vi "Error Converter (ErrCode or Status).vi"(0 "error code":u32, 11 "error in (no error)":errorcluster) -> (15 "error out":errorcluster)   [LabVIEW 2011, in "libMPSSE.lvlib"]
doc: "This VI generate the error description and error code from the dll error number."
uses:
  libMPSSE.lvlib
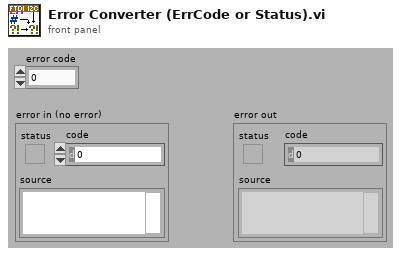
[diagram p1: front panel]
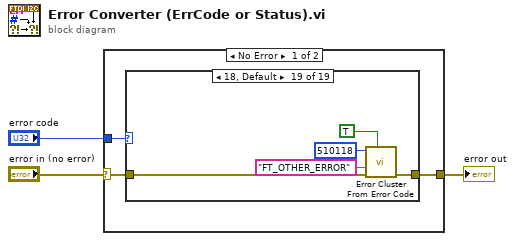
[diagram p0: block diagram]
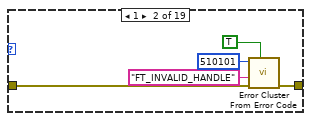
[diagram p3: hidden frame]
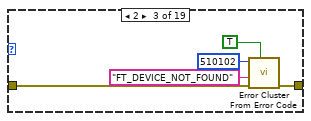
[diagram p4: hidden frame]
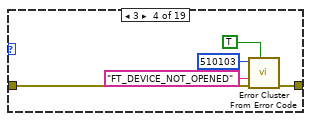
[diagram p5: hidden frame]
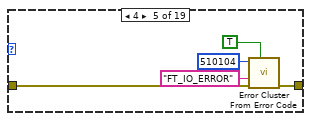
[diagram p6: hidden frame]
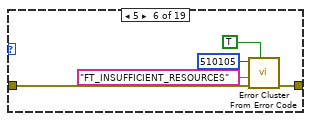
[diagram p7: hidden frame]
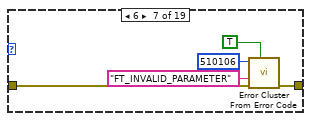
[diagram p8: hidden frame]
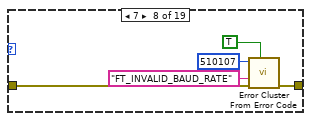
[diagram p9: hidden frame]
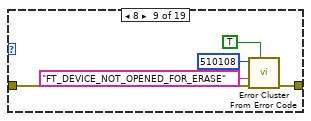
[diagram p10: hidden frame]
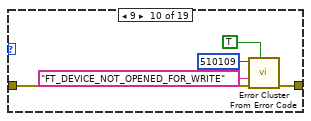
[diagram p11: hidden frame]
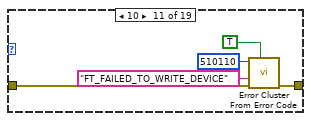
[diagram p12: hidden frame]
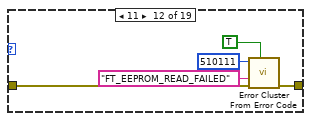
[diagram p13: hidden frame]
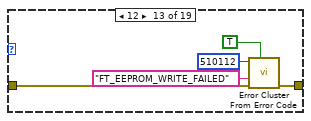
[diagram p14: hidden frame]
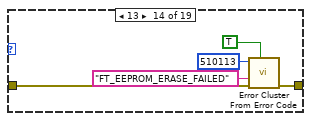
[diagram p15: hidden frame]
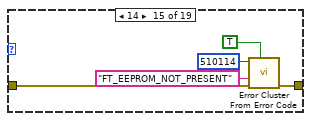
[diagram p16: hidden frame]
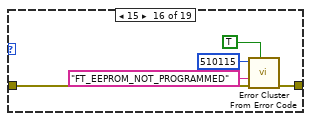
[diagram p17: hidden frame]
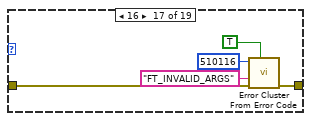
[diagram p18: hidden frame]
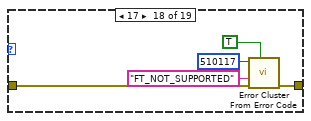
[diagram p19: hidden frame]
diagram:
  n1 = case shown="No Error" "error in (no error)" {
    selector: "error in (no error)" -> [w6 w98]
    tunnel: [w5 w98] -> w2
    tunnel: "error code" -> [w4 _]
    frame No Error {
      n2 = case shown="18, Default" w4 {
        tunnel: w6 -> [w7 w12 w17 w22 w27 w32 w37 w42 w47 w52 w57 w62 w67 w72 w77 w82 w87 w92 w97]
        tunnel: [w7 w11 w16 w21 w26 w31 w36 w41 w46 w51 w56 w61 w66 w71 w76 w81 w86 w91 w96] -> w5
        frame 0 {
        }
        frame 1 {
          n3 = call <vilib>:"Error Cluster From Error Code.vi"("show call chain? (False)"=TRUE, "error in (no error)"=w12, "error message (\"\")"="FT_INVALID_HANDLE", "error code (0)"=510101) -> ("error out"=w11:errorcluster)  [unwired: 5 in]
        }
        frame 2 {
          n4 = call <vilib>:"Error Cluster From Error Code.vi"("show call chain? (False)"=TRUE, "error in (no error)"=w17, "error message (\"\")"="FT_DEVICE_NOT_FOUND", "error code (0)"=510102) -> ("error out"=w16:errorcluster)  [unwired: 5 in]
        }
        frame 3 {
          n5 = call <vilib>:"Error Cluster From Error Code.vi"("show call chain? (False)"=TRUE, "error in (no error)"=w22, "error message (\"\")"="FT_DEVICE_NOT_OPENED", "error code (0)"=510103) -> ("error out"=w21:errorcluster)  [unwired: 5 in]
        }
        frame 4 {
          n6 = call <vilib>:"Error Cluster From Error Code.vi"("show call chain? (False)"=TRUE, "error in (no error)"=w27, "error message (\"\")"="FT_IO_ERROR", "error code (0)"=510104) -> ("error out"=w26:errorcluster)  [unwired: 5 in]
        }
        frame 5 {
          n7 = call <vilib>:"Error Cluster From Error Code.vi"("show call chain? (False)"=TRUE, "error in (no error)"=w32, "error message (\"\")"="FT_INSUFFICIENT_RESOURCES", "error code (0)"=510105) -> ("error out"=w31:errorcluster)  [unwired: 5 in]
        }
        frame 6 {
          n8 = call <vilib>:"Error Cluster From Error Code.vi"("show call chain? (False)"=TRUE, "error in (no error)"=w37, "error message (\"\")"="FT_INVALID_PARAMETER", "error code (0)"=510106) -> ("error out"=w36:errorcluster)  [unwired: 5 in]
        }
        frame 7 {
          n9 = call <vilib>:"Error Cluster From Error Code.vi"("show call chain? (False)"=TRUE, "error in (no error)"=w42, "error message (\"\")"="FT_INVALID_BAUD_RATE", "error code (0)"=510107) -> ("error out"=w41:errorcluster)  [unwired: 5 in]
        }
        frame 8 {
          n10 = call <vilib>:"Error Cluster From Error Code.vi"("show call chain? (False)"=TRUE, "error in (no error)"=w47, "error message (\"\")"="FT_DEVICE_NOT_OPENED_FOR_ERASE", "error code (0)"=510108) -> ("error out"=w46:errorcluster)  [unwired: 5 in]
        }
        frame 9 {
          n11 = call <vilib>:"Error Cluster From Error Code.vi"("show call chain? (False)"=TRUE, "error in (no error)"=w52, "error message (\"\")"="FT_DEVICE_NOT_OPENED_FOR_WRITE", "error code (0)"=510109) -> ("error out"=w51:errorcluster)  [unwired: 5 in]
        }
        frame 10 {
          n12 = call <vilib>:"Error Cluster From Error Code.vi"("show call chain? (False)"=TRUE, "error in (no error)"=w57, "error message (\"\")"="FT_FAILED_TO_WRITE_DEVICE", "error code (0)"=510110) -> ("error out"=w56:errorcluster)  [unwired: 5 in]
        }
        frame 11 {
          n13 = call <vilib>:"Error Cluster From Error Code.vi"("show call chain? (False)"=TRUE, "error in (no error)"=w62, "error message (\"\")"="FT_EEPROM_READ_FAILED", "error code (0)"=510111) -> ("error out"=w61:errorcluster)  [unwired: 5 in]
        }
        frame 12 {
          n14 = call <vilib>:"Error Cluster From Error Code.vi"("show call chain? (False)"=TRUE, "error in (no error)"=w67, "error message (\"\")"="FT_EEPROM_WRITE_FAILED", "error code (0)"=510112) -> ("error out"=w66:errorcluster)  [unwired: 5 in]
        }
        frame 13 {
          n15 = call <vilib>:"Error Cluster From Error Code.vi"("show call chain? (False)"=TRUE, "error in (no error)"=w72, "error message (\"\")"="FT_EEPROM_ERASE_FAILED", "error code (0)"=510113) -> ("error out"=w71:errorcluster)  [unwired: 5 in]
        }
        frame 14 {
          n16 = call <vilib>:"Error Cluster From Error Code.vi"("show call chain? (False)"=TRUE, "error in (no error)"=w77, "error message (\"\")"="FT_EEPROM_NOT_PRESENT", "error code (0)"=510114) -> ("error out"=w76:errorcluster)  [unwired: 5 in]
        }
        frame 15 {
          n17 = call <vilib>:"Error Cluster From Error Code.vi"("show call chain? (False)"=TRUE, "error in (no error)"=w82, "error message (\"\")"="FT_EEPROM_NOT_PROGRAMMED", "error code (0)"=510115) -> ("error out"=w81:errorcluster)  [unwired: 5 in]
        }
        frame 16 {
          n18 = call <vilib>:"Error Cluster From Error Code.vi"("show call chain? (False)"=TRUE, "error in (no error)"=w87, "error message (\"\")"="FT_INVALID_ARGS", "error code (0)"=510116) -> ("error out"=w86:errorcluster)  [unwired: 5 in]
        }
        frame 17 {
          n19 = call <vilib>:"Error Cluster From Error Code.vi"("show call chain? (False)"=TRUE, "error in (no error)"=w92, "error message (\"\")"="FT_NOT_SUPPORTED", "error code (0)"=510117) -> ("error out"=w91:errorcluster)  [unwired: 5 in]
        }
        frame 18, Default {
          n20 = call <vilib>:"Error Cluster From Error Code.vi"("show call chain? (False)"=TRUE, "error in (no error)"=w97, "error message (\"\")"="FT_OTHER_ERROR", "error code (0)"=510118) -> ("error out"=w96:errorcluster)  [unwired: 5 in]
        }
      }
    }
    frame Error {
    }
  }
  "error out" <- w2
